vi "EncoderSpeed3.vi"(8 "Cluster in":T1, 10 "Encoder 3 Controller":T3={"Sample time (uS)"=300000, "Reset"=FALSE}, 11 "error in (no error)":errorcluster) -> (0 "Cluster out":T1, 2 "Encoder 3 Indicator":T2, 3 "error out":errorcluster)   [LabVIEW 2014]
uses:
  controls/EncoderController.ctl
  controls/EncoderIndicator.ctl
  <vilib>/myRIO/Instrument Drivers/Onboard IO/Encoder/vis/Read.vi
  <vilib>/myRIO/Instrument Drivers/Onboard IO/Encoder/vis/Smart Open.vi
  <vilib>/Utility/error.llb/Error Cluster From Error Code.vi
  <vilib>/myRIO/Common/Instrument Driver Framework/myRIO v1.0/Encoder/vis/myRIO v1.0 Read Encoder.vi
  <vilib>/rvi/Arithmetic/AddSubMult/XNode/nirviSatArithmetic.xnode
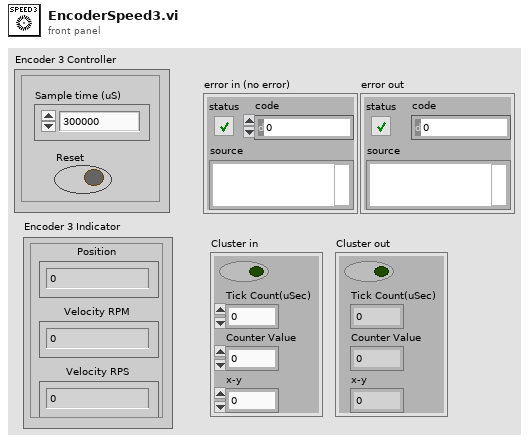
[diagram p1: front panel]
types:
  T1 = cluster{bool, "Tick Count(uSec)":u32, "Counter Value":i32, "x-y":i32}
  T2 = typedef "EncoderIndicator.ctl" = cluster{"Position":dbl, "Velocity RPM":dbl, "Velocity RPS":dbl}
  T3 = typedef "EncoderController.ctl" = cluster{"Sample time (uS)":u32, "Reset":bool}
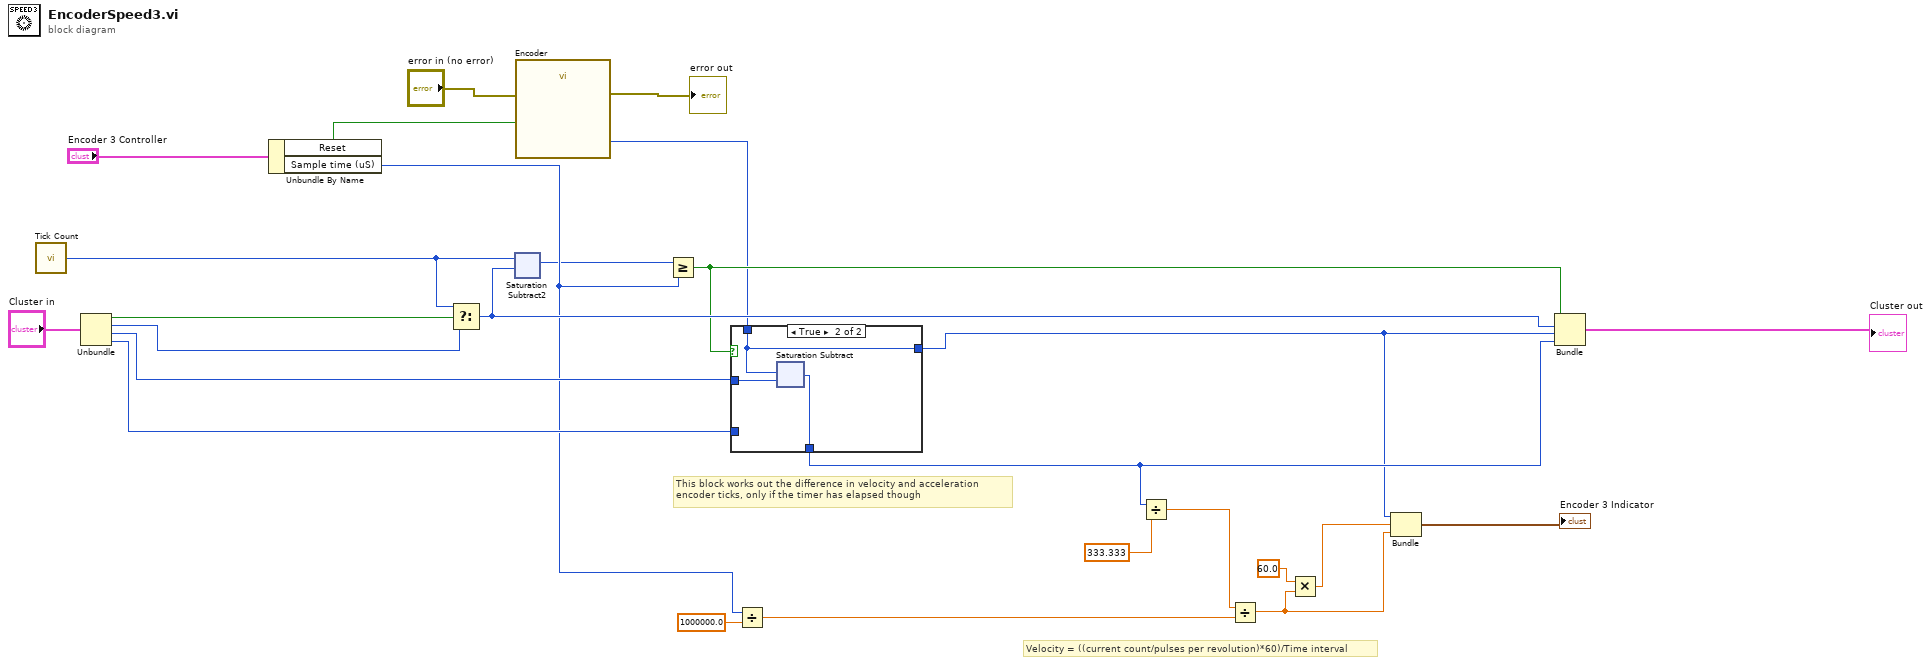
[diagram p0: block diagram]
diagram:
  # "Velocity = ((current count/pulses per revolution)*60)/Time interval"
  # "This block works out the difference in velocity and acceleration \nencoder ticks, only if the timer has elapsed though"
  n1 = call "Tick Count"() -> ("Tick Count(uSec)"=w14:u32)
  n2 = Unbundle("Cluster in") -> (w11:bool, "Tick Count(uSec)"=w12:u32, "Counter Value"=w13:i32, "x-y"=w19:i32)
  n3 = Unbundle By Name("Encoder 3 Controller") -> ("Reset"=w5:bool, "Sample time (uS)"=w6:u32)
  n4 = Select(t=w14, s=w11, f=w12) -> (s? t:f=w8:u32)
  n5 = xnode ("Saturation Subtract2")("x"=w14, "y"=w8) -> ("x-y"=w1:u32)
  n6 = call "Encoder"("Reset Counter"=w5, "error in (no error)"="error in (no error)") -> ("Counter Value"=w4:i32, "error out"=→"error out":errorcluster)  [unwired: 22 in, 2 out]
  n7 = Greater Or Equal?(x=w1, y=w6) -> (x >= y?=w7:bool)
  n8 = case shown="True" w7 {
    tunnel: w4 -> [_ w30]
    tunnel: w13 -> [w27 w31]
    tunnel: [w28 w29] -> w18
    tunnel: w19 -> [w28 _]
    tunnel: [w27 w30] -> w16
    frame False {
    }
    frame True {
      n9 = xnode ("Saturation Subtract")("x"=w30, "y"=w31) -> ("x-y"=w29:i32)
    }
  }
  n10 = Divide(x=w6, y=1000000.0) -> (x/y=w17:dbl)
  n11 = Divide(x=w18, y=333.333) -> (x/y=w20:dbl)
  n12 = Divide(x=w20, y=w17) -> (x/y=w21:dbl)
  n13 = Multiply(x=60.0 ("y"), y=w21) -> (x*y=w23:dbl)
  n14 = Bundle("Counter Value"=w16, w23, w21) -> (→"Encoder 3 Indicator":cluster{"Counter Value":i32, dbl, dbl})  [unwired: 1 in]
  n15 = Bundle(w7, "Tick Count(uSec)"=w8, "Counter Value"=w16, "x-y"=w18) -> (→"Cluster out":T1)  [unwired: 1 in]
